vi "Sub_Bounded_Regression.vi"(8 "Measuerd Frequency":dbl, 9 "Frequency":dbl[](array[numeric]), 10 "Pin":i32[](array[numeric]), 11 "Experiment in":T1) -> (2 "Pin estimate":i32, 3 "Position estimate":dbl)   [LabVIEW 2021]
uses:
  <vilib>/Analysis/baseanly.llb/Real A x B.vi
  <vilib>/Analysis/baseanly.llb/Real Inverse Matrix.vi
  <vilib>/Analysis/NI_AALBase.lvlib
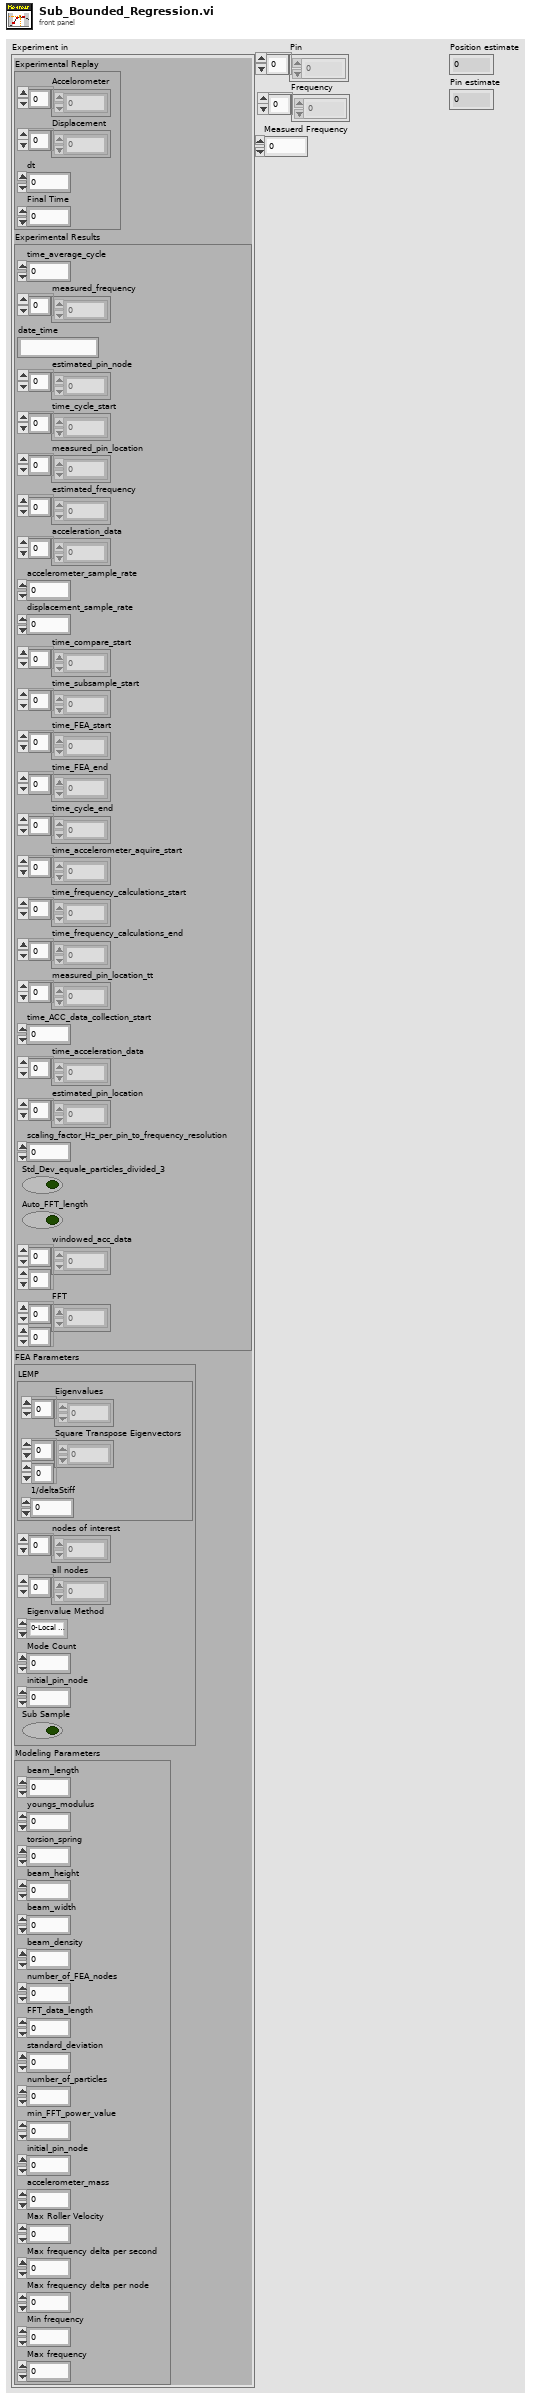
[diagram p1: front panel]
types:
  T1 = cluster{"Experimental Replay":cluster{"Accelorometer":dbl[], "Displacement":dbl[], "dt":dbl, "Final Time":dbl}, "Experimental Results":cluster{"time_average_cycle":dbl, "measured_frequency":dbl[], "date_time":string, "estimated_pin_node":i32[], "time_cycle_start":dbl[], "measured_pin_location":dbl[], "estimated_frequency":dbl[], "acceleration_data":dbl[], "accelerometer_sample_rate":dbl, "displacement_sample_rate":dbl, "time_compare_start":dbl[], "time_subsample_start":dbl[], "time_FEA_start":dbl[], "time_FEA_end":dbl[], "time_cycle_end":dbl[], "time_accelerometer_aquire_start":dbl[], "time_frequency_calculations_start":dbl[], "time_frequency_calculations_end":dbl[], "measured_pin_location_tt":dbl[], "time_ACC_data_collection_start":dbl, "time_acceleration_data":dbl[], "estimated_pin_location":dbl[], "scaling_factor_Hz_per_pin_to_frequency_resolution":dbl, "Std_Dev_equale_particles_divided_3":bool, "Auto_FFT_length":bool, "windowed_acc_data":dbl[][], "FFT":dbl[][]}, "FEA Parameters":cluster{"LEMP":cluster{"Eigenvalues":dbl[], "Square Transpose Eigenvectors":dbl[][], "1/deltaStiff":dbl}, "nodes of interest":i32[], "all nodes":i32[], "Eigenvalue Method":enum16{"0-Local Eigen Modification Procedure", "1-LabVIEW generalized eigenvalues", "2-LabVIEW M^-1K eigenvalues", "3-LabVIEW Cholesky Factorization", "4-Cholesky Factorization CPU SGL", "5-Cholesky Factorization CPU FXP", "6-Cholesky Factorization FPGA SGL", "7-Cholesky Factorization FPGA SGL SCL"}, "Mode Count":i32, "initial_pin_node":i32, "Sub Sample":bool}, "Modeling Parameters":cluster{"beam_length":dbl, "youngs_modulus":dbl, "torsion_spring":dbl, "beam_height":dbl, "beam_width":dbl, "beam_density":dbl, "number_of_FEA_nodes":i32, "FFT_data_length":i32, "standard_deviation":dbl, "number_of_particles":i32, "min_FFT_power_value":dbl, "initial_pin_node":i32, "accelerometer_mass":dbl, "Max Roller Velocity":dbl, "Max frequency delta per second":dbl, "Max frequency delta per node":dbl, "Min frequency":dbl, "Max frequency":dbl}}
  T2 = typedef "NI_Matrix.lvlib/RealMatrix.ctl" = dbl[][]
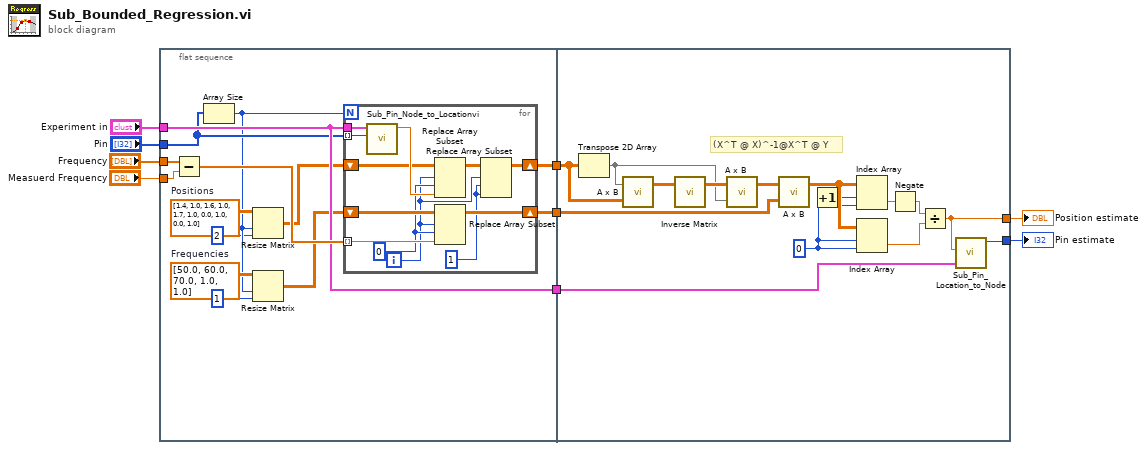
[diagram p0: block diagram]
diagram:
  n1 = flat-sequence {
    tunnel: [w23] -> w9
    tunnel: [w22] -> w8
    tunnel: [w18] -> w6
    tunnel: "Measuerd Frequency" -> [w20]
    tunnel: "Frequency" -> [w19]
    tunnel: "Pin" -> [w17]
    tunnel: "Experiment in" -> [w18]
    tunnel: w9 -> [w50]
    tunnel: w8 -> [w45]
    tunnel: [w38] -> w7
    tunnel: w6 -> [w37]
    tunnel: [w36] -> w5
    frame #0 {
      w14 = dbl[][] [[50.0], [60.0], [70.0], [1.0], [1.0]]  # Frequencies
      w16 = dbl[][] [[1.4, 1.0], [1.6, 1.0], [1.7, 1.0], [0.0, 1.0], [0.0, 1.0]]  # Positions
      n2 = Subtract(x=w19, y=w20) -> (x-y=w21:dbl[])
      n3 = Array Size(array=w17) -> (size(s)=w12:i32)
      n4 = Resize Matrix(1:2 ("number of columns"), 2:w12, 4:w16) -> (0:w15:dbl[][])
      n5 = Resize Matrix(1:1, 2:w12, 4:w14) -> (0:w13:dbl[][])
      n6 = for {
        N: w12 -> [_]
        tunnel: w17 -> [w35] mode=indexing
        tunnel: w18 -> [w34]
        tunnel: w21 -> [w32] mode=indexing
        shift-right: [w28] -> w22
        shift-left: w13 -> [w30]
        shift-right: [w26] -> w23
        shift-left: w15 -> [w31]
        i -> [w25]
        w24 = 1 ("disabled index (row)")
        w29 = 0 ("disabled index (col)")
        n7 = call "Sub_Pin_Node_to_Locationvi.vi"("Node"=w35, "Experiment in"=w34) -> ("Pin location"=w33:dbl)  [unwired: 9 in]
        n8 = Replace Array Subset(array=w31, new element=w33, index (row)=w25, index (col)=w29) -> (w27:dbl[][])
        n9 = Replace Array Subset(array=w30, new element=w32, index (row)=w25, index (col)=w29) -> (w28:dbl[][])
        n10 = Replace Array Subset(array=w27, new element=w24, index (row)=w25, index (col)=w24) -> (w26:dbl[][])
      }
    }
    frame #1 {
      w41 = 0 ("index (row)")
      # "(X^T @ X)^-1@X^T @ Y"
      n11 = Transpose 2D Array(2D array=w50) -> (transposed array=w47:dbl[][])
      n12 = call-poly <vilib>:"A x B.vi"("B"=w50, "A"=w47) -> ("A x B"=w49:T2)  [unwired: 1 out]
      n13 = call-poly <vilib>:"Inverse Matrix.vi"("Input Matrix"=w49) -> ("Inverse Matrix"=w48:T2)  [unwired: 1 in, 1 out]
      n14 = call-poly <vilib>:"A x B.vi"("B"=w47, "A"=w48) -> ("A x B"=w46:T2)  [unwired: 1 out]
      n15 = call-poly <vilib>:"A x B.vi"("B"=w45, "A"=w46) -> ("A x B"=w44:T2)  [unwired: 1 out]
      n16 = Increment(x=w41) -> (x+1=w42:i32)
      n17 = Index Array(array=w44, index (row)=w42, index (col)=w41) -> (element=w40:dbl)
      n18 = Index Array(array=w44, index (row)=w41, index (col)=w41) -> (element=w43:dbl)
      n19 = Negate(x=w40) -> (-x=w39:dbl)
      n20 = Divide(x=w39, y=w43) -> (x/y=w38:dbl)
      n21 = call "Sub_Pin_Location_to_Node.vi"("Pin Location"=w38, "Experiment in"=w37) -> ("DOF of Interest"=w36:i32)  [unwired: 9 in]
    }
  }
  "Position estimate" <- w7
  "Pin estimate" <- w5
